vi "TemplateGUITAF_CastUIEvent.vi"(11 "UIEvent":T2) -> (1 "Data":variant, 2 "ApplicationGUIOut":refnum<class "TemplateGUITAF.lvclass">, 3 "UiEventNames":T1)   [LabVIEW 2021, in "TemplateGUITAF.lvlib" / "TemplateGUITAF.lvclass"]
uses:
  TemplateGUITAF.lvclass
  TemplateGUITAF_UiCallBackEvents.ctl
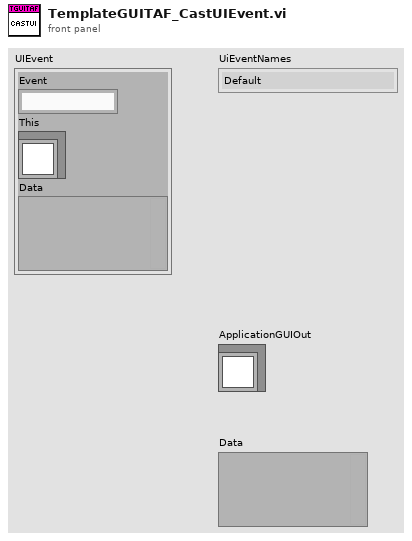
[diagram p1: front panel]
types:
  T1 = typedef "TemplateGUITAF.lvlib/TemplateGUITAF.lvclass/TemplateGUITAF_UiCallBackEvents.ctl" = enum16{"Default", "PersistentDataUpdated"}
  T2 = cluster{"Event":string, "This":refnum<class>, "Data":variant}
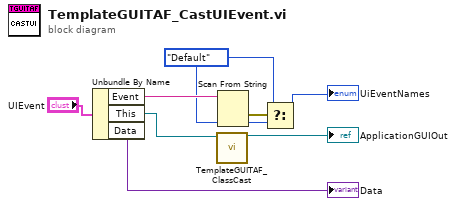
[diagram p0: block diagram]
diagram:
  w2 = TemplateGUITAF_UiCallBackEvents."Default" ("UiEventNames")
  n1 = Unbundle By Name("UIEvent") -> ("Event"=w6:string, "This"=w5:refnum<class>, "Data"=→"Data":variant)
  n2 = call "TemplateGUITAF_ClassCast.vi"("TemplateGUITAF in"=w5) -> ("TemplateGUITAF out"=→"ApplicationGUIOut":refnum<class "TemplateGUITAF.lvclass">)  [unwired: 10 in]
  n3 = Scan From String(input string=w6, default 1=w2) -> (error out=w9:errorcluster, output 1=w4:T1)  [unwired: 3 in, 2 out]
  n4 = Select(t=w2, s=w9, f=w4) -> (s? t:f=→"UiEventNames":T1)
